vi "Sprinkler.vi"(5 "Stop":bool, 6 "Start":bool, 7 "Zone Setup Array":cluster{"Zone Selector":T1, "Timing":dbl}[](array[cluster]), 8 "Setup":bool, 9 "Run Selector":bool, 10 "Water Pressure Sensor (%)":dbl(slide)=100.0 scale=0.0..100.0, 11 "Rain Sensor":bool) -> (0 "error out":errorcluster, 3 "Zone Indicators":T2)   [LabVIEW 2018]
doc: "Use this template to build a standard state machine design pattern. Each state executes code and determines which state to transition to. Contrast this design pattern with the User Interface Event Handler pattern, in which code executes in response to user actions. Contrast this design pattern also with the Queued Message Handler pattern, in which each message handling code can queue zero or more new messages."
uses:
  Controls/Zone Selector.ctl
  Controls/StateMachineStates.ctl
  Controls/Timing.ctl
  <vilib>/Utility/file.llb/Read Delimited Spreadsheet (string).vi
panel:
  out "Controller Status":string
  # "CLD Sprinkler Control v1.0"
  # "Continuous\n\nSingle"
  # "Simulation Controls"
  # "Rain\n\nNo Rain"
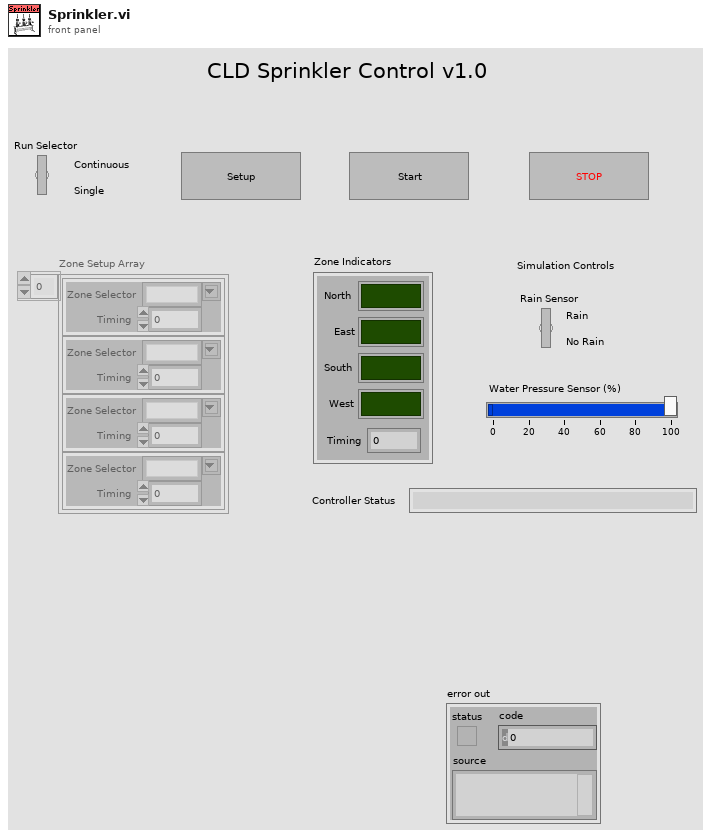
[diagram p1: front panel]
types:
  T1 = typedef "Zone Selector.ctl" = string
  T2 = cluster{"North":bool, "East":bool, "South":bool, "West":bool, "Timing":i32}
  T3 = typedef "StateMachineStates.ctl" = enum16{"Initialize", "Wait for User Input", "Setup", "Zone North", "Zone East", "Zone South", "Zone West", "Low Pressure", "Rain", "Stop"}
  T4 = enum8{"Enabled", "Disabled", "Disabled and Grayed Out"}
  T5 = typedef "Timing.ctl" = enum16{"Reset Time", "Time Elapsed"}
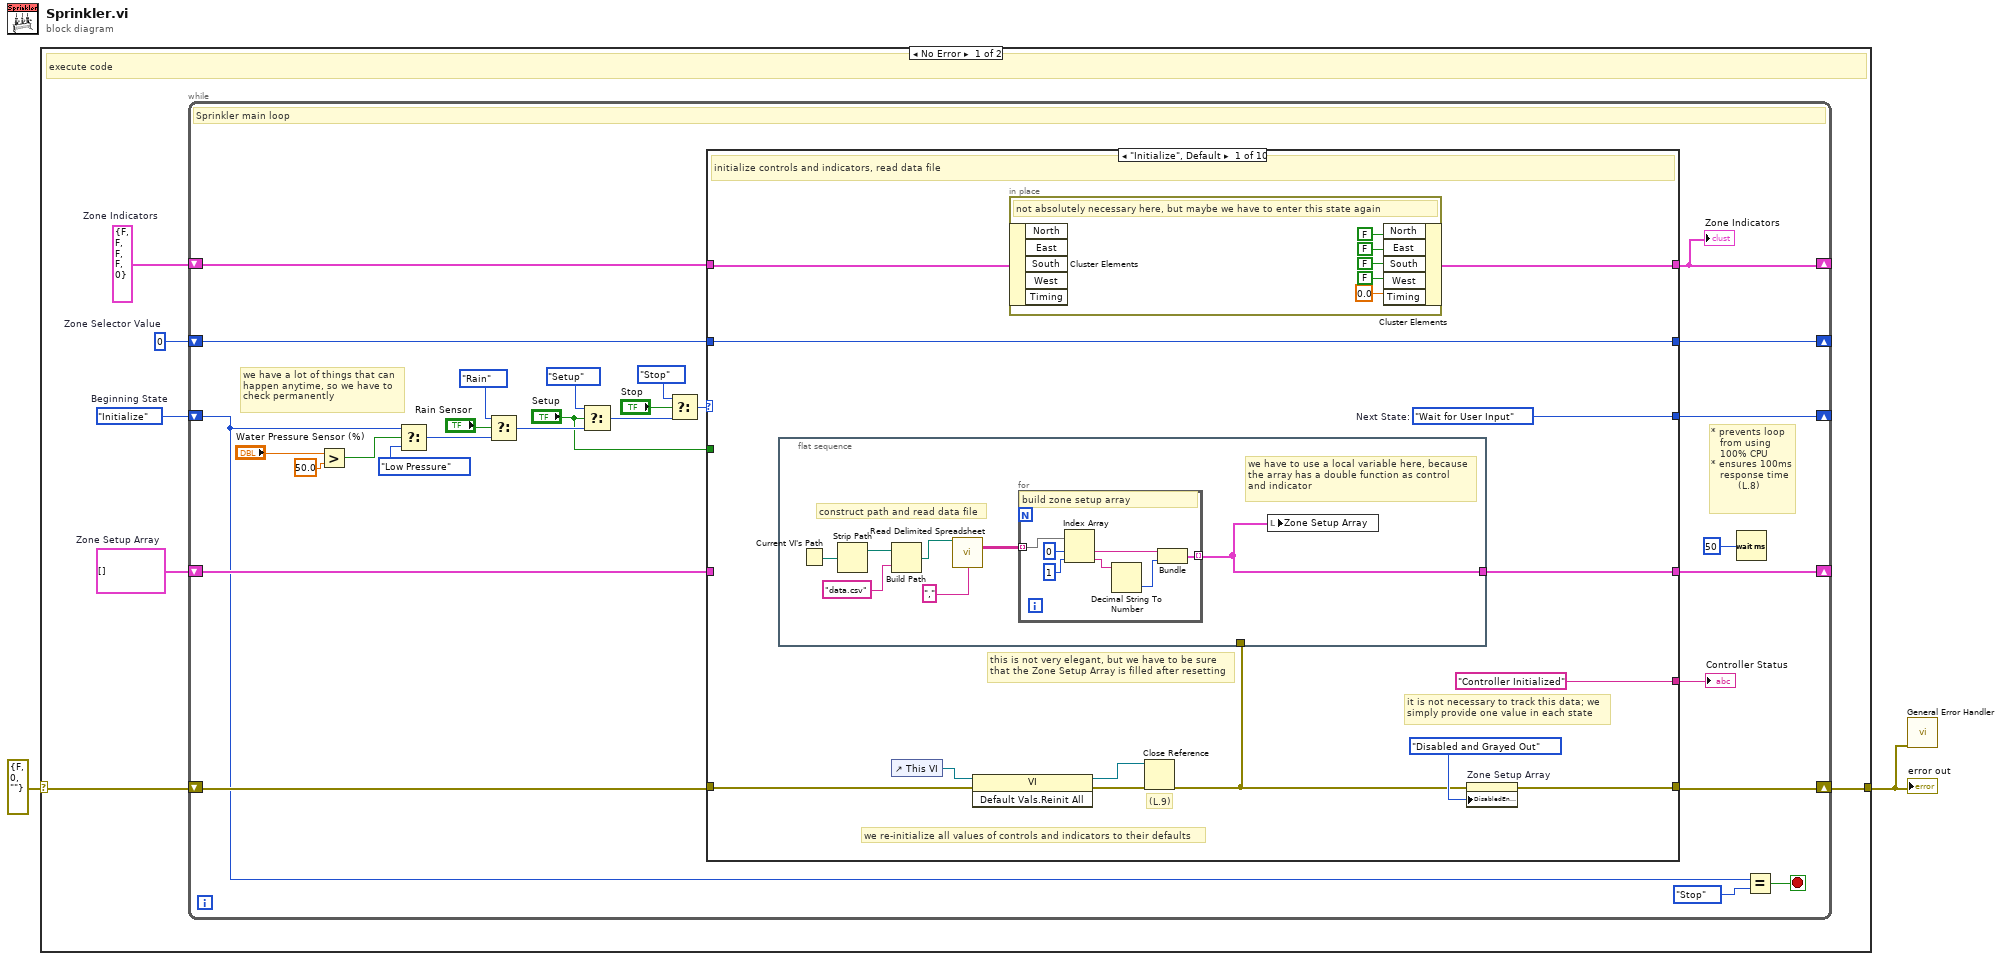
[diagram p0: block diagram]
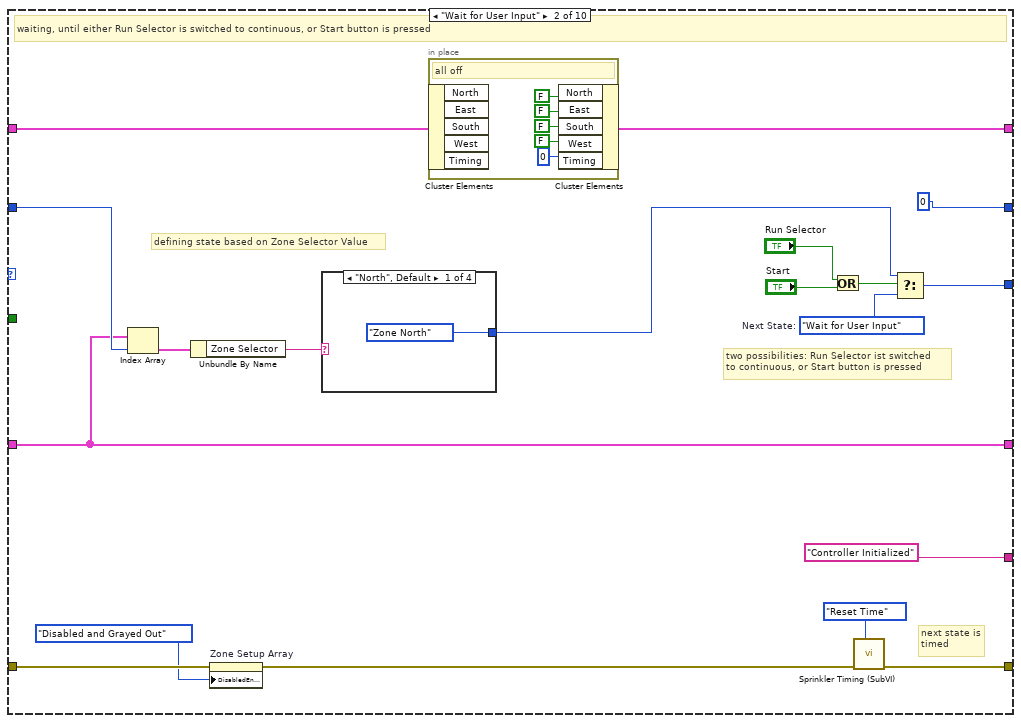
[diagram p2: hidden frame]
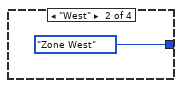
[diagram p3: hidden frame]
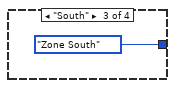
[diagram p4: hidden frame]
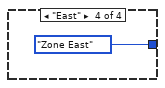
[diagram p5: hidden frame]
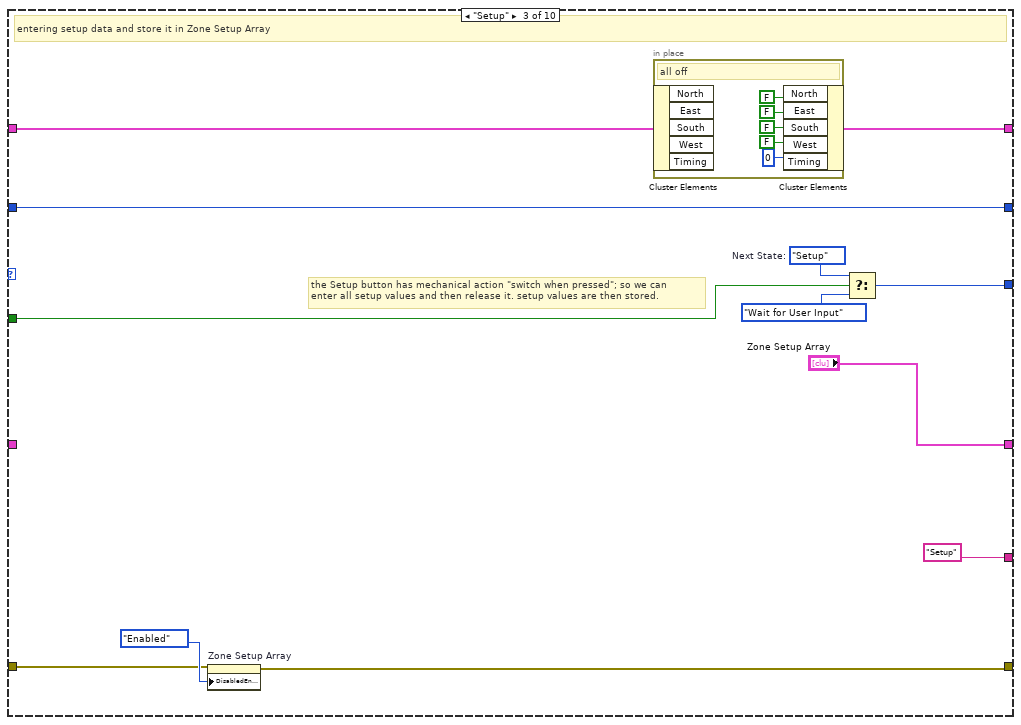
[diagram p6: hidden frame]
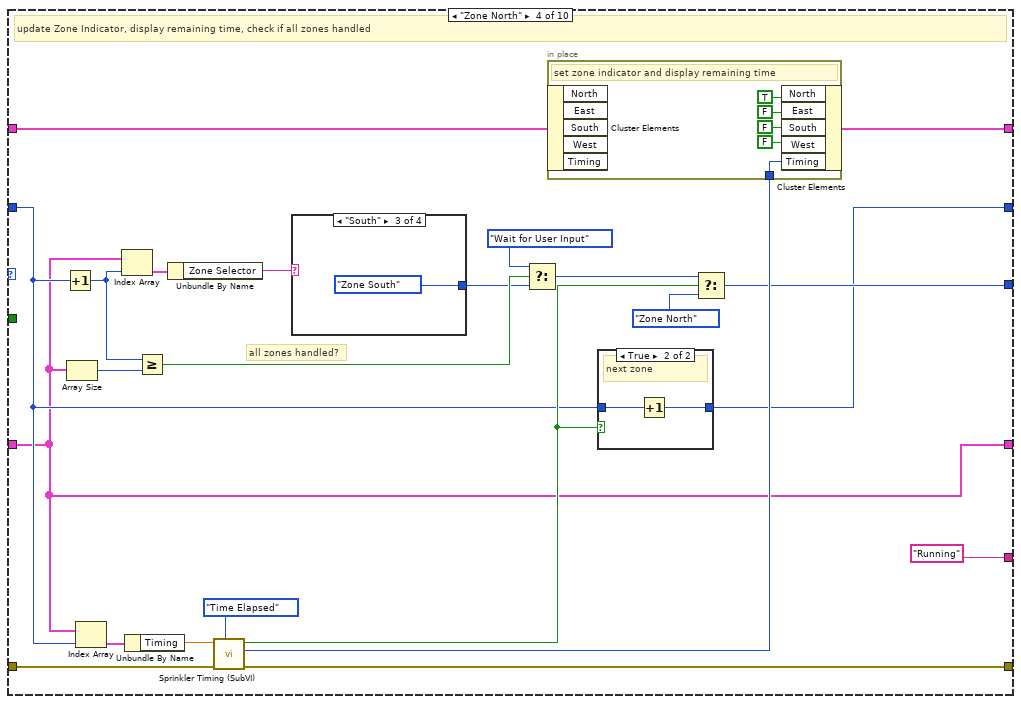
[diagram p7: hidden frame]
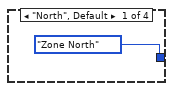
[diagram p9: hidden frame]
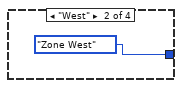
[diagram p10: hidden frame]
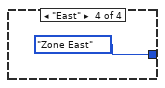
[diagram p11: hidden frame]
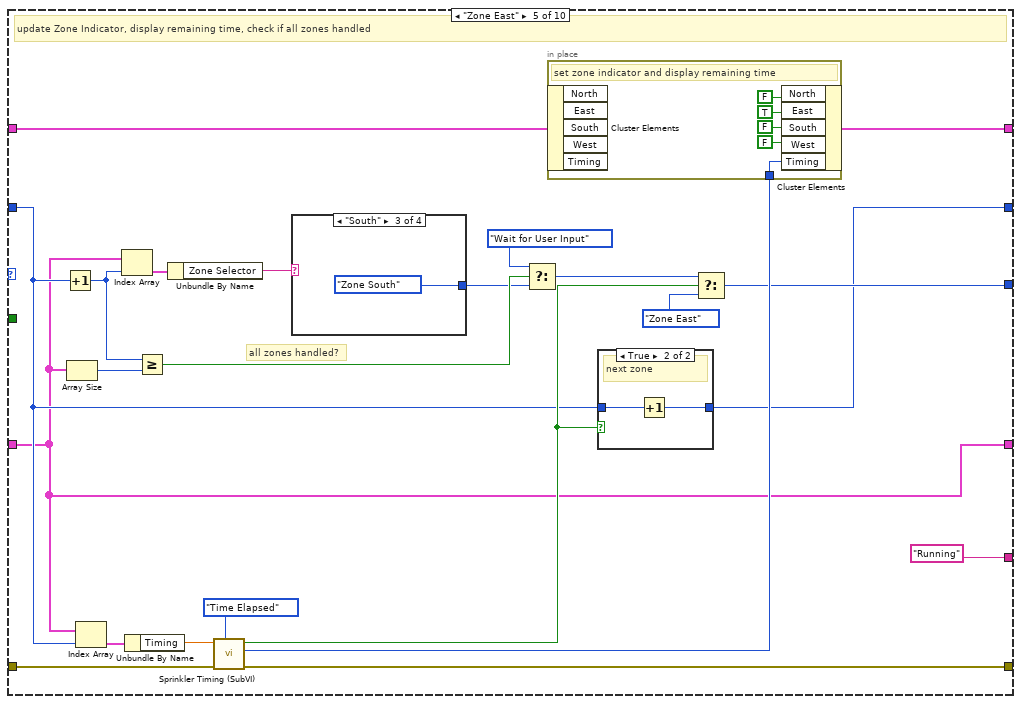
[diagram p12: hidden frame]
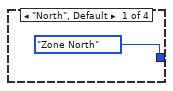
[diagram p14: hidden frame]
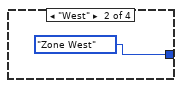
[diagram p15: hidden frame]
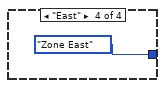
[diagram p16: hidden frame]
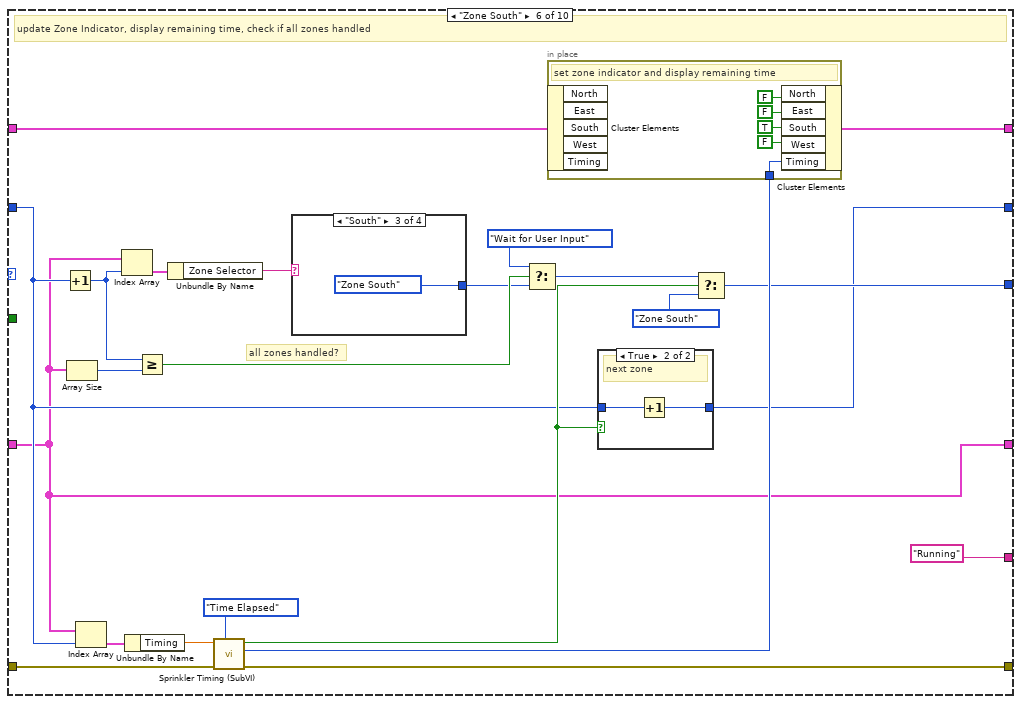
[diagram p17: hidden frame]
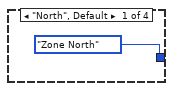
[diagram p19: hidden frame]
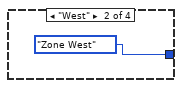
[diagram p20: hidden frame]
diagram:
  n1 = case shown="No Error" errorcluster {"status"=FALSE, "code"=0, "source"=""} ("error in (no error)") {
    selector: errorcluster {"status"=FALSE, "code"=0, "source"=""} ("error in (no error)") -> [w5 w308]
    tunnel: [w6 w308] -> w1
    frame No Error {
      w3 = cluster{"Zone Selector":T1, "Timing":dbl}[] []  # Zone Setup Array
      w4 = 0  # Zone Selector Value
      w7 = T2 {"North"=FALSE, "East"=FALSE, "South"=FALSE, "West"=FALSE, "Timing"=0}  # Zone Indicators
      w8 = StateMachineStates."Initialize"  # Beginning State
      # "execute code"
      n2 = while {
        shift-right: [w9] -> _
        shift-left: w8 -> [w11]
        shift-right: [w32] -> _
        shift-left: w7 -> [w33]
        shift-right: [w31] -> w6
        shift-left: w5 -> [w30]
        shift-right: [w26] -> _
        shift-left: w4 -> [w27]
        shift-right: [w12] -> _
        shift-left: w3 -> [w28]
        stop <- w25 stop-if-true
        # "we have a lot of things that can\nhappen anytime, so we have to\ncheck permanently"
        # "* prevents loop\n   from using\n   100% CPU\n* ensures 100ms\n   response time\n         (L.8)"
        # "Sprinkler main loop"
        n3 = Greater?(x="Water Pressure Sensor (%)", y=50.0) -> (0:w22:bool)
        n4 = Select(t=w11, s=w22, f=StateMachineStates."Low Pressure") -> (s? t:f=w17:T3)
        n5 = Select(t=StateMachineStates."Rain" ("f"), s="Rain Sensor", f=w17) -> (s? t:f=w15:T3)
        n6 = Select(t=StateMachineStates."Setup" ("Beginning State"), s="Setup", f=w15) -> (s? t:f=w14:T3)
        n7 = Select(t=StateMachineStates."Stop" ("Beginning State"), s="Stop", f=w14) -> (s? t:f=w10:T3)
        n8 = case shown="\"Initialize\", Default" w10 {
          tunnel: [w49 w87 w101 w128 w163 w198 w233 StateMachineStates."Stop" ("Next State") w268 w289] -> w9
          tunnel: ["Controller Initialized" "Controller Initialized" "Setup" "Running" "Running" "Running" "Running" "Stopped" "Low Water Pressure" "Rain"] -> w34
          tunnel: [w41 w70 w108 w131 w166 w201 w236 w257 w269 w290] -> w32
          tunnel: w33 -> [w40 w69 w107 w132 w167 w202 w237 w258 w270 w291]
          tunnel: w30 -> [w45 w74 w99 w136 w171 w206 w241 w256 w272 w293]
          tunnel: [w43 w82 w98 w116 w151 w186 w221 w256 w273 w294] -> w31
          tunnel: w28 -> [_ w71 _ w114 w149 w184 w219 w254 w266 w287]
          tunnel: w27 -> [w39 w83 w105 w118 w153 w188 w223 w255 w267 w288]
          tunnel: [w39 0 w105 w117 w152 w187 w222 w255 w267 w288] -> w26
          tunnel: "Setup" -> [_ _ w104 _ _ _ _ _ _ _]
          tunnel: [w38 w71 "Zone Setup Array" w114 w149 w184 w219 w254 w266 w287] -> w12
          frame "Initialize", Default {
            w49 = StateMachineStates."Wait for User Input"  # Next State:
            # "this is not very elegant, but we have to be sure\nthat the Zone Setup Array is filled after resetting"
            # "it is not necessary to track this data; we \nsimply provide one value in each state"
            # "we re-initialize all values of controls and indicators to their defaults"
            # "(L.9)"
            # "initialize controls and indicators, read data file"
            n9 = flat-sequence {
              tunnel: [w56] -> w38
              tunnel: w37 -> [_]
              frame #0 {
                # "we have to use a local variable here, because\nthe array has a double function as control\nand indicator"
                # "construct path and read data file"
                n10 = Current VI's Path() -> (path=w53:path)
                n11 = Strip Path(path=w53) -> (stripped path=w55:path)  [unwired: 1 out]
                n12 = Build Path(base path=w55, name or relative path="data.csv") -> (appended path=w52:path)
                n13 = call-poly <vilib>:"Read Delimited Spreadsheet.vi"("file path (dialog if empty)"=w52, "delimiter (\\t)"="," ("delimiter (\\t)")) -> ("all rows"=w50:string[][])  [unwired: 8 in, 5 out]
                n14 = for {
                  tunnel: w50 -> [w62] mode=indexing
                  tunnel: [w60] -> w56 mode=indexing
                  # "build zone setup array"
                  n15 = Index Array(array=w62, index #1=0 ("index"), index #2=1 ("index")) -> (element #1=w61:string, element #2=w57:string)
                  n16 = Decimal String To Number(string=w57) -> (number=w59:i32)  [unwired: 2 in, 1 out]
                  n17 = Bundle("String"=w61, w59) -> (w60:cluster{"String":string, i32})  [unwired: 1 in]
                }
                n18 = local write "Zone Setup Array"(w56) -> ()
              }
            }
            n19 = control-ref of="This VI"() -> (w48:refnum<vi>)
            n20 = invoke class="VI" method="Default Vals.Reinit All"(reference=w48, error in=w45) -> (reference out=w47:refnum<vi>, error out=w46:errorcluster)  [unwired: 1 in, 1 out]
            n21 = in-place {
              # "not absolutely necessary here, but maybe we have to enter this state again"
              n22 = in-place-cluster #1(w40) -> ()  [unwired: 5 out]
              n23 = in-place-cluster #1("North"=FALSE, "East"=FALSE, "South"=FALSE, "West"=FALSE, "Timing"=0.0) -> (w41:T2)
            }
            n24 = Close Reference(reference=w47, error in (no error)=w46) -> (error out=w37:errorcluster)
            n25 = property on="Zone Setup Array" class="Arr (strict)"(error in=w37, "DisabledEnum"=T4."Disabled and Grayed Out" ("Disabled")) -> (error out=w43:errorcluster)  [unwired: 1 in, 1 out]
          }
          frame "Wait for User Input" {
            w75 = StateMachineStates."Wait for User Input"  # Next State:
            # "next state is\ntimed"
            # "two possibilities: Run Selector ist switched \nto continuous, or Start button is pressed"
            # "defining state based on Zone Selector Value"
            # "waiting, until either Run Selector is switched to continuous, or Start button is pressed"
            n26 = Index Array "Index Array"(array=w71, index=w83) -> (element=w85:cluster{"Zone Selector":T1, "Timing":dbl})
            n27 = Unbundle By Name(w85) -> ("Zone Selector"=w86:T1)
            n28 = property on="Zone Setup Array" class="Arr (strict)"(error in=w74, "DisabledEnum"=T4."Disabled and Grayed Out" ("Disabled")) -> (error out=w73:errorcluster)  [unwired: 1 in, 1 out]
            n29 = case shown="\"North\", Default" w86 {
              tunnel: [StateMachineStates."Zone North" ("Beginning State") StateMachineStates."Zone West" ("Beginning State") StateMachineStates."Zone South" ("Beginning State") StateMachineStates."Zone East" ("Beginning State")] -> w84
              frame "North", Default {
              }
              frame "West" {
              }
              frame "South" {
              }
              frame "East" {
              }
            }
            n30 = in-place {
              # "all off"
              n31 = in-place-cluster #2(w69) -> ()  [unwired: 5 out]
              n32 = in-place-cluster #2("North"=FALSE, "East"=FALSE, "South"=FALSE, "West"=FALSE, "Timing"=0) -> (w70:T2)
            }
            n33 = Or(x="Run Selector", y="Start") -> (x .or. y?=w76:bool)
            n34 = call "Sprinkler Timing (SubVI).vi"("Function"=Timing."Reset Time" ("Enum"), "error in (no error)"=w73) -> ("error out"=w82:errorcluster)  [unwired: 7 in, 2 out]
            n35 = Select(t=w84, s=w76, f=w75) -> (s? t:f=w87:T3)
          }
          frame "Setup" {
            w102 = StateMachineStates."Setup"  # Next State:
            # "the Setup button has mechanical action \"switch when pressed\"; so we can \nenter all setup values and then release it. setup values are then stored."
            # "entering setup data and store it in Zone Setup Array"
            n36 = property on="Zone Setup Array" class="Arr (strict)"(error in=w99, "DisabledEnum"=T4."Enabled" ("Disabled")) -> (error out=w98:errorcluster)  [unwired: 1 in, 1 out]
            n37 = in-place {
              # "all off"
              n38 = in-place-cluster #3(w107) -> ()  [unwired: 5 out]
              n39 = in-place-cluster #3("North"=FALSE, "East"=FALSE, "South"=FALSE, "West"=FALSE, "Timing"=0) -> (w108:T2)
            }
            n40 = Select(t=w102, s=w104, f=StateMachineStates."Wait for User Input") -> (s? t:f=w101:T3)
          }
          frame "Zone North" {
            # "all zones handled?"
            # "update Zone Indicator, display remaining time, check if all zones handled"
            n41 = Increment(x=w118) -> (x+1=w124:i32)
            n42 = Array Size(array=w114) -> (size(s)=w125:i32)
            n43 = Index Array "Index Array"(array=w114, index=w118) -> (element=w135:cluster{"Zone Selector":T1, "Timing":dbl})
            n44 = Index Array "Index Array"(array=w114, index=w124) -> (element=w127:cluster{"Zone Selector":T1, "Timing":dbl})
            n45 = Unbundle By Name(w135) -> ("Timing"=w134:dbl)
            n46 = Greater Or Equal?(x=w124, y=w125) -> (x >= y?=w123:bool)
            n47 = Unbundle By Name(w127) -> ("Zone Selector"=w126:T1)
            n48 = call "Sprinkler Timing (SubVI).vi"("Function"=Timing."Time Elapsed" ("Enum"), "error in (no error)"=w136, "Time to Wait (s)"=w134) -> ("error out"=w116:errorcluster, "Remaining Time"=w130:i32, "Time elapsed ?"=w119:bool)  [unwired: 6 in]
            n49 = case shown="\"South\"" w126 {
              tunnel: [StateMachineStates."Zone North" ("Beginning State") StateMachineStates."Zone West" ("Beginning State") StateMachineStates."Zone South" ("Beginning State") StateMachineStates."Zone East" ("Beginning State")] -> w122
              frame "North", Default {
              }
              frame "West" {
              }
              frame "South" {
              }
              frame "East" {
              }
            }
            n50 = Select(t=StateMachineStates."Wait for User Input" ("Beginning State"), s=w123, f=w122) -> (s? t:f=w121:T3)
            n51 = in-place {
              in-place-border: w130 -> [w144]
              # "set zone indicator and display remaining time"
              n52 = in-place-cluster #4(w132) -> ()  [unwired: 5 out]
              n53 = in-place-cluster #4("North"=TRUE, "East"=FALSE, "South"=FALSE, "West"=FALSE, "Timing"=w144) -> (w131:T2)
            }
            n54 = case shown="True" w119 {
              tunnel: w118 -> [w137 w139]
              tunnel: [w137 w138] -> w117
              frame False {
                # "same zone"
              }
              frame True {
                # "next zone"
                n55 = Increment(x=w139) -> (x+1=w138:i32)
              }
            }
            n56 = Select(t=w121, s=w119, f=StateMachineStates."Zone North" ("Beginning State")) -> (s? t:f=w128:T3)
          }
          frame "Zone East" {
            # "all zones handled?"
            # "update Zone Indicator, display remaining time, check if all zones handled"
            n57 = Increment(x=w153) -> (x+1=w159:i32)
            n58 = Array Size(array=w149) -> (size(s)=w160:i32)
            n59 = Index Array "Index Array"(array=w149, index=w153) -> (element=w170:cluster{"Zone Selector":T1, "Timing":dbl})
            n60 = Index Array "Index Array"(array=w149, index=w159) -> (element=w162:cluster{"Zone Selector":T1, "Timing":dbl})
            n61 = Unbundle By Name(w170) -> ("Timing"=w169:dbl)
            n62 = Greater Or Equal?(x=w159, y=w160) -> (x >= y?=w158:bool)
            n63 = Unbundle By Name(w162) -> ("Zone Selector"=w161:T1)
            n64 = call "Sprinkler Timing (SubVI).vi"("Function"=Timing."Time Elapsed" ("Enum"), "error in (no error)"=w171, "Time to Wait (s)"=w169) -> ("error out"=w151:errorcluster, "Remaining Time"=w165:i32, "Time elapsed ?"=w154:bool)  [unwired: 6 in]
            n65 = case shown="\"South\"" w161 {
              tunnel: [StateMachineStates."Zone North" ("Beginning State") StateMachineStates."Zone West" ("Beginning State") StateMachineStates."Zone South" ("Beginning State") StateMachineStates."Zone East" ("Beginning State")] -> w157
              frame "North", Default {
              }
              frame "West" {
              }
              frame "South" {
              }
              frame "East" {
              }
            }
            n66 = Select(t=StateMachineStates."Wait for User Input" ("Beginning State"), s=w158, f=w157) -> (s? t:f=w156:T3)
            n67 = in-place {
              in-place-border: w165 -> [w179]
              # "set zone indicator and display remaining time"
              n68 = in-place-cluster #5(w167) -> ()  [unwired: 5 out]
              n69 = in-place-cluster #5("North"=FALSE, "East"=TRUE, "South"=FALSE, "West"=FALSE, "Timing"=w179) -> (w166:T2)
            }
            n70 = case shown="True" w154 {
              tunnel: w153 -> [w172 w174]
              tunnel: [w172 w173] -> w152
              frame False {
                # "same zone"
              }
              frame True {
                # "next zone"
                n71 = Increment(x=w174) -> (x+1=w173:i32)
              }
            }
            n72 = Select(t=w156, s=w154, f=StateMachineStates."Zone East" ("Beginning State")) -> (s? t:f=w163:T3)
          }
          frame "Zone South" {
            # "all zones handled?"
            # "update Zone Indicator, display remaining time, check if all zones handled"
            n73 = Increment(x=w188) -> (x+1=w194:i32)
            n74 = Array Size(array=w184) -> (size(s)=w195:i32)
            n75 = Index Array "Index Array"(array=w184, index=w188) -> (element=w205:cluster{"Zone Selector":T1, "Timing":dbl})
            n76 = Index Array "Index Array"(array=w184, index=w194) -> (element=w197:cluster{"Zone Selector":T1, "Timing":dbl})
            n77 = Unbundle By Name(w205) -> ("Timing"=w204:dbl)
            n78 = Greater Or Equal?(x=w194, y=w195) -> (x >= y?=w193:bool)
            n79 = Unbundle By Name(w197) -> ("Zone Selector"=w196:T1)
            n80 = call "Sprinkler Timing (SubVI).vi"("Function"=Timing."Time Elapsed" ("Enum"), "error in (no error)"=w206, "Time to Wait (s)"=w204) -> ("error out"=w186:errorcluster, "Remaining Time"=w200:i32, "Time elapsed ?"=w189:bool)  [unwired: 6 in]
            n81 = case shown="\"South\"" w196 {
              tunnel: [StateMachineStates."Zone North" ("Beginning State") StateMachineStates."Zone West" ("Beginning State") StateMachineStates."Zone South" ("Beginning State") StateMachineStates."Zone East" ("Beginning State")] -> w192
              frame "North", Default {
              }
              frame "West" {
              }
              frame "South" {
              }
              frame "East" {
              }
            }
            n82 = Select(t=StateMachineStates."Wait for User Input" ("Beginning State"), s=w193, f=w192) -> (s? t:f=w191:T3)
            n83 = in-place {
              in-place-border: w200 -> [w214]
              # "set zone indicator and display remaining time"
              n84 = in-place-cluster #6(w202) -> ()  [unwired: 5 out]
              n85 = in-place-cluster #6("North"=FALSE, "East"=FALSE, "South"=TRUE, "West"=FALSE, "Timing"=w214) -> (w201:T2)
            }
            n86 = case shown="True" w189 {
              tunnel: w188 -> [w207 w209]
              tunnel: [w207 w208] -> w187
              frame False {
                # "same zone"
              }
              frame True {
                # "next zone"
                n87 = Increment(x=w209) -> (x+1=w208:i32)
              }
            }
            n88 = Select(t=w191, s=w189, f=StateMachineStates."Zone South" ("Beginning State")) -> (s? t:f=w198:T3)
          }
          frame "Zone West" {
            # "all zones handled?"
            # "update Zone Indicator, display remaining time, check if all zones handled"
            n89 = Increment(x=w223) -> (x+1=w229:i32)
            n90 = Array Size(array=w219) -> (size(s)=w230:i32)
            n91 = Index Array "Index Array"(array=w219, index=w223) -> (element=w240:cluster{"Zone Selector":T1, "Timing":dbl})
            n92 = Index Array "Index Array"(array=w219, index=w229) -> (element=w232:cluster{"Zone Selector":T1, "Timing":dbl})
            n93 = Unbundle By Name(w240) -> ("Timing"=w239:dbl)
            n94 = Greater Or Equal?(x=w229, y=w230) -> (x >= y?=w228:bool)
            n95 = Unbundle By Name(w232) -> ("Zone Selector"=w231:T1)
            n96 = call "Sprinkler Timing (SubVI).vi"("Function"=Timing."Time Elapsed" ("Enum"), "error in (no error)"=w241, "Time to Wait (s)"=w239) -> ("error out"=w221:errorcluster, "Remaining Time"=w235:i32, "Time elapsed ?"=w224:bool)  [unwired: 6 in]
            n97 = case shown="\"South\"" w231 {
              tunnel: [StateMachineStates."Zone North" ("Beginning State") StateMachineStates."Zone West" ("Beginning State") StateMachineStates."Zone South" ("Beginning State") StateMachineStates."Zone East" ("Beginning State")] -> w227
              frame "North", Default {
              }
              frame "West" {
              }
              frame "South" {
              }
              frame "East" {
              }
            }
            n98 = Select(t=StateMachineStates."Wait for User Input" ("Beginning State"), s=w228, f=w227) -> (s? t:f=w226:T3)
            n99 = in-place {
              in-place-border: w235 -> [w249]
              # "set zone indicator and display remaining time"
              n100 = in-place-cluster #7(w237) -> ()  [unwired: 5 out]
              n101 = in-place-cluster #7("North"=FALSE, "East"=FALSE, "South"=FALSE, "West"=TRUE, "Timing"=w249) -> (w236:T2)
            }
            n102 = case shown="True" w224 {
              tunnel: w223 -> [w242 w244]
              tunnel: [w242 w243] -> w222
              frame False {
                # "same zone"
              }
              frame True {
                # "next zone"
                n103 = Increment(x=w244) -> (x+1=w243:i32)
              }
            }
            n104 = Select(t=w226, s=w224, f=StateMachineStates."Zone West" ("Beginning State")) -> (s? t:f=w233:T3)
          }
          frame "Stop" {
            # "just to be sure that the\nprogram is really stopped"
            # "stopping the program"
            n105 = in-place {
              # "all off"
              n106 = in-place-cluster #8(w258) -> ()  [unwired: 5 out]
              n107 = in-place-cluster #8("North"=FALSE, "East"=FALSE, "South"=FALSE, "West"=FALSE, "Timing"=0) -> (w257:T2)
            }
          }
          frame "Low Pressure" {
            # "next state is\ntimed"
            # "we check the water pressure outside the case, so we simply have to load the zone that continues after restoring the pressure"
            n108 = Index Array "Index Array"(array=w266, index=0) -> (element=w275:cluster{"Zone Selector":T1, "Timing":dbl})
            n109 = Unbundle By Name(w275) -> ("Zone Selector"=w274:T1)
            n110 = case shown="\"South\"" w274 {
              tunnel: [StateMachineStates."Zone North" ("Beginning State") StateMachineStates."Zone West" ("Beginning State") StateMachineStates."Zone South" ("Beginning State") StateMachineStates."Zone East" ("Beginning State")] -> w268
              frame "North", Default {
              }
              frame "West" {
              }
              frame "South" {
              }
              frame "East" {
              }
            }
            n111 = in-place {
              # "also here all off"
              n112 = in-place-cluster #9(w270) -> ()  [unwired: 5 out]
              n113 = in-place-cluster #9("North"=FALSE, "East"=FALSE, "South"=FALSE, "West"=FALSE, "Timing"=0) -> (w269:T2)
            }
            n114 = call "Sprinkler Timing (SubVI).vi"("Function"=Timing."Reset Time" ("Enum"), "error in (no error)"=w272) -> ("error out"=w273:errorcluster)  [unwired: 7 in, 2 out]
          }
          frame "Rain" {
            # "next state is\ntimed"
            # "we check the rain sensor outside the case, so we simply have to load the zone that continues after rain has stopped"
            n115 = Index Array "Index Array"(array=w287, index=0) -> (element=w296:cluster{"Zone Selector":T1, "Timing":dbl})
            n116 = Unbundle By Name(w296) -> ("Zone Selector"=w295:T1)
            n117 = case shown="\"South\"" w295 {
              tunnel: [StateMachineStates."Zone North" ("Beginning State") StateMachineStates."Zone West" ("Beginning State") StateMachineStates."Zone South" ("Beginning State") StateMachineStates."Zone East" ("Beginning State")] -> w289
              frame "North", Default {
              }
              frame "West" {
              }
              frame "South" {
              }
              frame "East" {
              }
            }
            n118 = in-place {
              # "also here all off"
              n119 = in-place-cluster #10(w291) -> ()  [unwired: 5 out]
              n120 = in-place-cluster #10("North"=FALSE, "East"=FALSE, "South"=FALSE, "West"=FALSE, "Timing"=0) -> (w290:T2)
            }
            n121 = call "Sprinkler Timing (SubVI).vi"("Function"=Timing."Reset Time" ("Enum"), "error in (no error)"=w293) -> ("error out"=w294:errorcluster)  [unwired: 7 in, 2 out]
          }
        }
        "Zone Indicators" <- w32
        "Controller Status" <- w34
        n122 = Wait (ms)(milliseconds to wait=u32 50) -> ()  [unwired: 1 out]
        n123 = Equal?(x=w11, y=StateMachineStates."Stop" ("States")) -> (x = y?=w25:bool)
      }
    }
    frame Error {
      # "do  nothing"
    }
  }
  "error out" <- w1
  n124 = call <vilib>:"General Error Handler.vi"("error in (no error)"=w1) -> ()  [unwired: 10 in, 5 out]
